vi "IP_CheckIfValid.vi"(11 "IP":string) -> (3 "Valid IP":bool)   [LabVIEW 2022 SP3, in "hse-network.lvlib"]
doc: "Check if the string input is a valid IP address\n\n____\nHAMPEL SOFTWARE ENGINEERING v3.8.0 (2023-12-18 14:41)"
uses:
  hse-network.lvlib
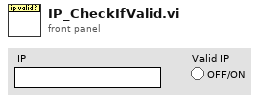
[diagram p1: front panel]
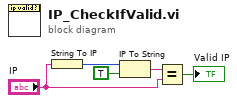
[diagram p0: block diagram]
diagram:
  n1 = String To IP(1:"IP") -> (0:w1:u32)
  n2 = IP To String(1:TRUE, 2:w1) -> (0:w3:string)
  n3 = Equal?(x=w3, y="IP") -> (x = y?=→"Valid IP":bool)
